vi "FT_Read_Byte_Data.vi"(0 "Handle":u64, 1 "Bytes To Read":u32) -> (2 "FT_Status":u32, 3 "Read Data":u8[](array[numeric]), 4 "Bytes Read":u32)   [LabVIEW 2025, in "FT.lvlib"]
uses:
  FT.lvlib
  FTD2XX.dll
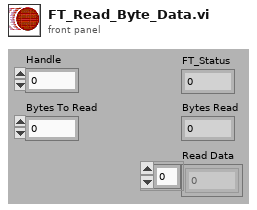
[diagram p1: front panel]
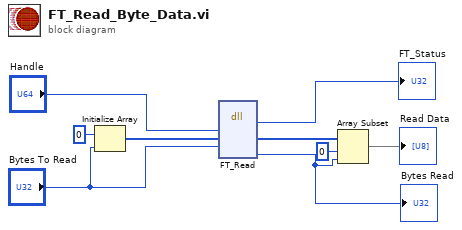
[diagram p0: block diagram]
diagram:
  n1 = Initialize Array(u8 0 ("element"), "Bytes To Read") -> (w7:u8[])
  n2 = dll-call lib="FTD2XX.dll" fn="FT_Read"("Handle"="Handle", "Buffer"=w7, "BytesToRead"="Bytes To Read") -> ("FT_Status"=→"FT_Status":u32, "Buffer"=w4:u8[], "BytesReturned"=w2:u32)  [unwired: 6 in, 2 out]
  "Bytes Read" <- w2
  n3 = Array Subset(array=w4, index=0, length=w2) -> (→"Read Data":u8[])
